vi "Test Listbox.vi"() -> ()   [LabVIEW 2020, in "ListBoxTests.lvlib"]
uses:
  ListBoxTests.lvlib
  <vilib>/addons/_JKI Toolkits/Caraya/classes/Test Suite/Define Test Suite (JUnit Report).vi
  <vilib>/SLL Drona/APIs/Stimulus/VI/MakeVIFrontMost.vi
  <vilib>/SLL Drona/APIs/Get/GetControlRef/GetControlRefByPath.vi
  <vilib>/SLL Drona/APIs/Stimulus/ControlValue/ValueSignalByPathString.vi
  <vilib>/SLL Drona/APIs/Assert/AssertControlValue/Equal.vi
  <vilib>/SLL Drona/APIs/Stimulus/VI/CloseVI.vi
  <vilib>/Utility/error.llb/Error Cluster From Error Code.vi
  <vilib>/ErrorRing/Error Ring.xnode
  <vilib>/addons/_JKI Toolkits/Caraya/classes/Test Suite/Test Suite.lvclass
  <vilib>/addons/_JKI Toolkits/Caraya/classes/Test/Test.lvclass
  <vilib>/SLL Drona/Drona.lvlib
  <vilib>/Wiresmith Technology/G CLI/CLI Class/CLI.lvclass
  <vilib>/SLL Drona/APIs/Stimulus/ControlValue/ControlValue.lvlib
  <vilib>/SLL Drona/APIs/Get/GetControlRef/GetControlRef.lvlib
  <vilib>/SLL Drona/APIs/Stimulus/VI/VI.lvlib
  <vilib>/SLL Drona/APIs/Assert/AssertControlValue/AssertControlValue.lvlib
  <vilib>/addons/_JKI Toolkits/Caraya/classes/Assert/Assert.lvclass
panel:
  out "Error out":errorcluster
  in  "Error in":errorcluster
  # "LISTBOX TEST"
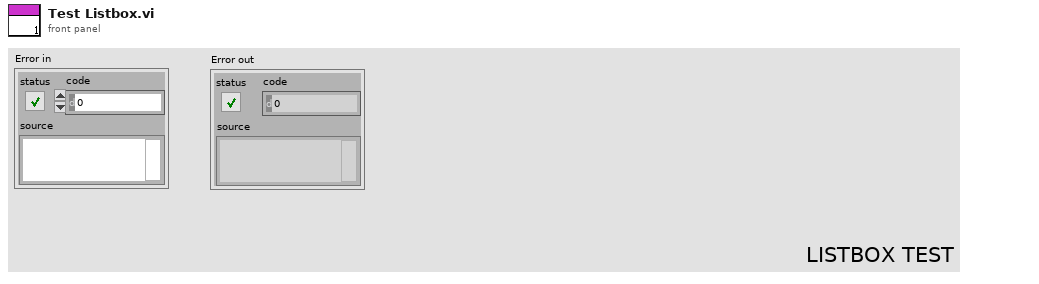
[diagram p1: front panel]
types:
  T1 = typedef "LVRectTypeDef.ctl" = cluster{"Left":i16, "Top":i16, "Right":i16, "Bottom":i16}
  T2 = typedef "LVPositionTypeDef.ctl" = cluster{"Left":i32, "Top":i32}
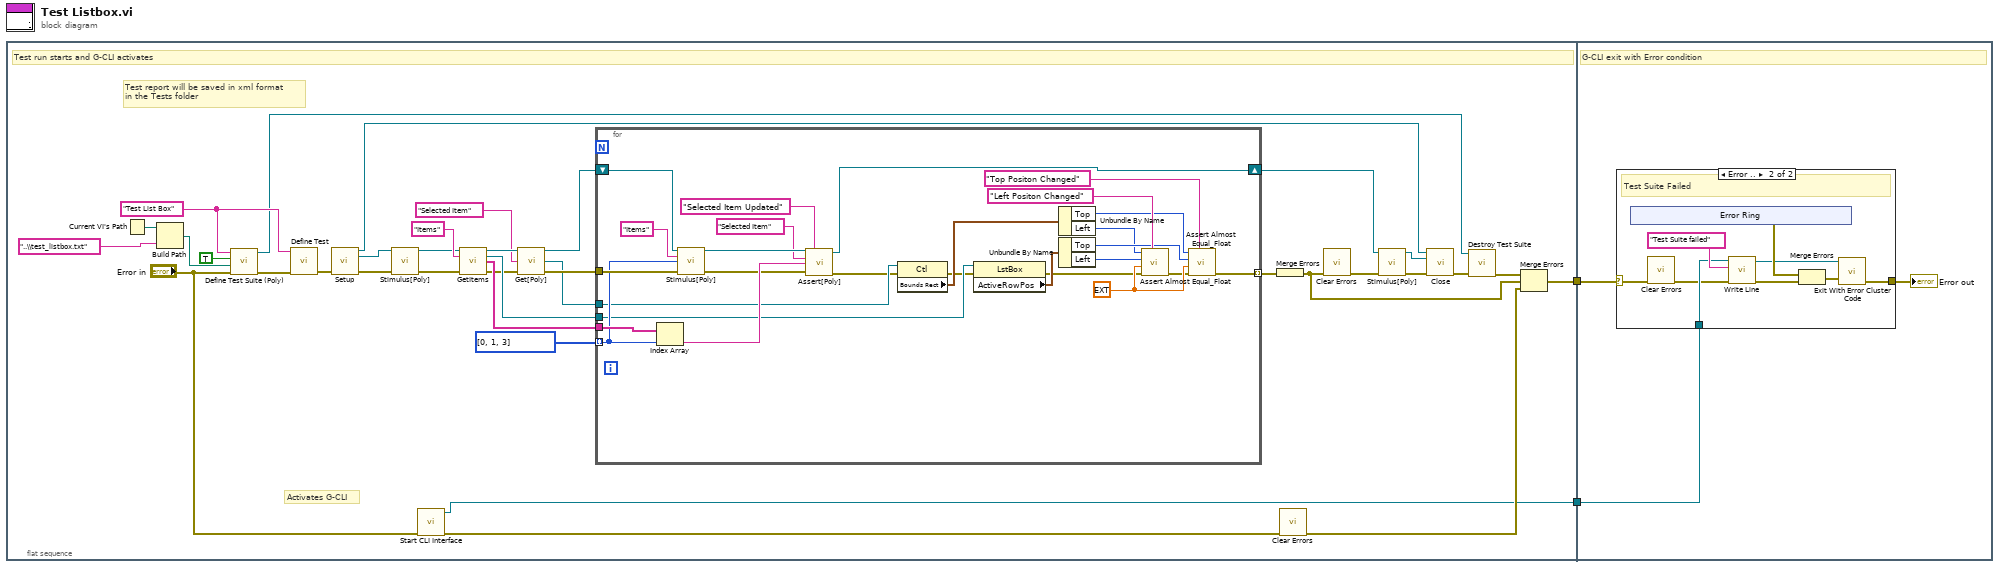
[diagram p0: block diagram]
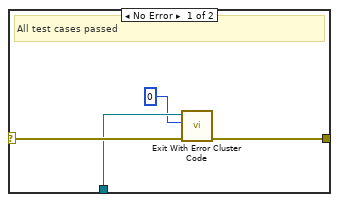
[diagram p2: hidden frame]
diagram:
  n1 = flat-sequence {
    tunnel: [w22] -> w2
    tunnel: [w21] -> w1
    tunnel: w2 -> [w68]
    tunnel: w1 -> [w67]
    frame #0 {
      w34 = "Test List Box" ("Label (VI Title)")
      # "Activates G-CLI"
      # "Test report will be saved in xml format\nin the Tests folder"
      # "Test run starts and G-CLI activates"
      n2 = Current VI's Path() -> (path=w33:path)
      n3 = Build Path(base path=w33, name or relative path="..\\test_listbox.txt") -> (appended path=w31:path)
      n4 = call-poly <vilib>:"Define Test Suite (Poly).vi"("error in (no error)"="Error in", "Report Path"=w31, "Interactive"=TRUE, "Label (VI Title)"=w34) -> ("error out"=w35:errorcluster, "Test Suite"=w28:refnum<class "Test Suite.lvclass">)  [unwired: 5 in, 1 out]
      n5 = call <vilib>:"Define Test.vi"("error in (no error)"=w35, "Label (VI Title)"=w34) -> ("error out"=w38:errorcluster)  [unwired: 8 in, 1 out]
      n6 = call <vilib>:"Setup.vi"("error in"=w38) -> ("Application Ref"=w7:refnum<vi>, "VI Reference Out"=w6:refnum<vi>, "error out"=w4:errorcluster)  [unwired: 12 in]
      n7 = call-poly <vilib>:"Stimulus[Poly].vi"("VI Reference In"=w6, "error in"=w4) -> ("VI Reference Out"=w5:refnum<vi>, "error out"=w3:errorcluster)  [unwired: 12 in]
      n8 = call <vilib>:"Start CLI Interface.vi"("error in (no error)"="Error in") -> ("error out"=w24:errorcluster, "CLI out"=w21:refnum<class "CLI.lvclass">)  [unwired: 7 in, 2 out]
      n9 = call "GetItems.vi"("VI Reference In"=w5, "Control Path"="Items", "error In"=w3) -> ("VI Reference Out"=w14:refnum<vi>, "LstBox Refnum"=w19:refnum<vi>, "Items[]"=w18:string[], "error out"=w16:errorcluster)  [unwired: 9 in]
      n10 = call-poly <vilib>:"Get[Poly].vi"("VI Reference In"=w14, "Control Path"="Selected Item", "error In"=w16) -> ("VI Reference Out"=w13:refnum<vi>, "Ctl Refnum"=w12:refnum<vi>, "error out"=w15:errorcluster)  [unwired: 10 in]
      n11 = for {
        tunnel: w15 -> [w64]
        tunnel: w19 -> [w55]
        tunnel: w18 -> [w60]
        shift-right: [w52] -> w8
        shift-left: w13 -> [w63]
        tunnel: i32[] [0, 1, 3] -> [w59] mode=indexing
        tunnel: w12 -> [w54]
        tunnel: [w53] -> w11 mode=indexing
        w47 = ext 5.0 ("Tolerance")
        n12 = Index Array(array=w60, index=w59) -> (element=w58:string)
        n13 = call-poly <vilib>:"Stimulus[Poly].vi"("VI Reference In"=w63, "Control Path"="Items", "Value (Signaling)"=w59, "error in"=w64) -> ("VI Reference Out"=w62:refnum<vi>, "error out"=w56:errorcluster)  [unwired: 10 in]
        n14 = call-poly <vilib>:"Assert[Poly].vi"("VI Reference In"=w62, "Test Label"="Selected Item Updated", "Control Path"="Selected Item", "Control Value"=w58, "Error In"=w56) -> ("VI Reference Out"=w52:refnum<vi>, "Error Out"=w51:errorcluster)  [unwired: 9 in]
        n15 = property class="Ctl"(reference=w54, error in=w51) -> (error out=w40:errorcluster, "Bounds Rect"=w48:T1)  [unwired: 1 out]
        n16 = property class="LstBox"(reference=w55, error in=w40) -> (error out=w39:errorcluster, "ActiveRowPos"=w49:T2)  [unwired: 1 out]
        n17 = Unbundle By Name(w48) -> ("Top"=w45:i16, "Left"=w41:i16)
        n18 = Unbundle By Name(w49) -> ("Top"=w44:i32, "Left"=w42:i32)
        n19 = call <vilib>:"Assert Almost Equal_Float.vi"("Label"="Left Positon Changed" ("Test Label"), "error in (no error)"=w39, "Tolerance"=w47, "Y"=w42, "X"=w41) -> ("error out"=w43:errorcluster)  [unwired: 5 in, 1 out]
        n20 = call <vilib>:"Assert Almost Equal_Float.vi"("Label"="Top Positon Changed" ("Test Label"), "error in (no error)"=w43, "Tolerance"=w47, "Y"=w44, "X"=w45) -> ("error out"=w53:errorcluster)  [unwired: 5 in, 1 out]
      }
      n21 = Merge Errors(w11) -> (w10:errorcluster)
      n22 = call <vilib>:"Clear Errors.vi"("error in (no error)"=w24) -> ("error out"=w23:errorcluster)  [unwired: 5 in, 1 out]
      n23 = call <vilib>:"Clear Errors.vi"("error in (no error)"=w10) -> ("error out"=w25:errorcluster)  [unwired: 5 in, 1 out]
      n24 = call-poly <vilib>:"Stimulus[Poly].vi"("VI Reference In"=w8, "error in"=w25) -> ("VI Reference Out"=w37:refnum<vi>, "error out"=w36:errorcluster)  [unwired: 12 in]
      n25 = call <vilib>:"Close.vi"("Application Ref"=w7, "VI Reference"=w37, "error in"=w36) -> ("error out"=w29:errorcluster)  [unwired: 12 in]
      n26 = call-dynamic "Destroy Test Suite.vi"("error in (no error)"=w29, "Test Suite in"=w28) -> ("error out"=w26:errorcluster)  [unwired: 8 in, 1 out]
      n27 = Merge Errors(w26, w10, w23) -> (w22:errorcluster)
    }
    frame #1 {
      # "G-CLI exit with Error condition"
      n28 = case shown="Error .." w68 {
        selector: w68 -> [w72 w76]
        tunnel: w67 -> [w71 w74]
        tunnel: [w69 w81] -> w66
        frame No Error {
          # "All test cases passed"
          n29 = call <vilib>:"Exit With Error Cluster Code.vi"("error in (no error)"=w72, "No Error Code (0)"=0, "CLI in"=w71) -> ("error out"=w69:errorcluster)  [unwired: 8 in]
        }
        frame Error {
          # "Test Suite Failed"
          n30 = xnode "Error Ring"() -> ("error out"=w78:errorcluster)
          n31 = call <vilib>:"Clear Errors.vi"("error in (no error)"=w76) -> ("error out"=w73:errorcluster)  [unwired: 5 in, 1 out]
          n32 = call <vilib>:"Write Line.vi"("error in (no error)"=w73, "Text to Write"="Test Suite failed", "CLI in"=w74) -> ("error out"=w77:errorcluster, "CLI out"=w75:refnum<class "CLI.lvclass">)  [unwired: 7 in]
          n33 = Merge Errors(w78, w77) -> (w79:errorcluster)
          n34 = call <vilib>:"Exit With Error Cluster Code.vi"("error in (no error)"=w79, "CLI in"=w75) -> ("error out"=w81:errorcluster)  [unwired: 9 in]
        }
      }
      "Error out" <- w66
    }
  }
